vi "Diode_Control_Panel.vi"(11 "IP Address of Remote Device":string="196.254.31.200") -> ()   [LabVIEW 2020]
panel:
  in  "Visualization Tab Control":enum32{"Trace", "Metrics", "None"}(tab)
  out "Diode Trace":waveform(dbl)[](graph)
  out "Reduced Mean Signal, One Point = One Shot":dbl[](graph)
  out "(For your Reference: ) Query Sent to Device":string
  in  "Zero Time":bool
  out "Settable Device Keywords":string[](array[string])
  out "Live Readback Values":string[](array[string])
  in  "Set All":bool
  in  "Set Values\n(Fully empty cells will not be set)":string[](array[string])
  out "Live Responses":string[](array[string])
  out "Non-Settable Device Keywords":string[](array[string])
  in  "Disconnect":bool
  # "Diode Control Panel"
  # "General control panel to facilitate setup of diode, setting times, verifying quality of metrics."
  # "VI Instructions\n\n1. Make sure you know the Device IP Address.\n2. From Windows command prompt, confirm ping to IP address.\n3. Type the correct device IP address into this VI.\n3. Run this VI. *Note:* Only one TCP connection to the device's SCPI-like server can run at a time.\n4. When finished, disconnect safely from the device via the \"Disconnect\" toggle button. (Not the Abort button).\n\nCreated by Scott Feister on July 19, 2022.\nUpdated back panel details July 28, 2022."
  # "1. Resets the trigger count to zero.\n2. Transmits this system's current time."
  # "Settings *ARE NOT SAVED TO DEVICE* and are lost on device reset! Write them down!"
  # "Select the \"None\" tab to help other items update more quickly, and to save network bandwidth."
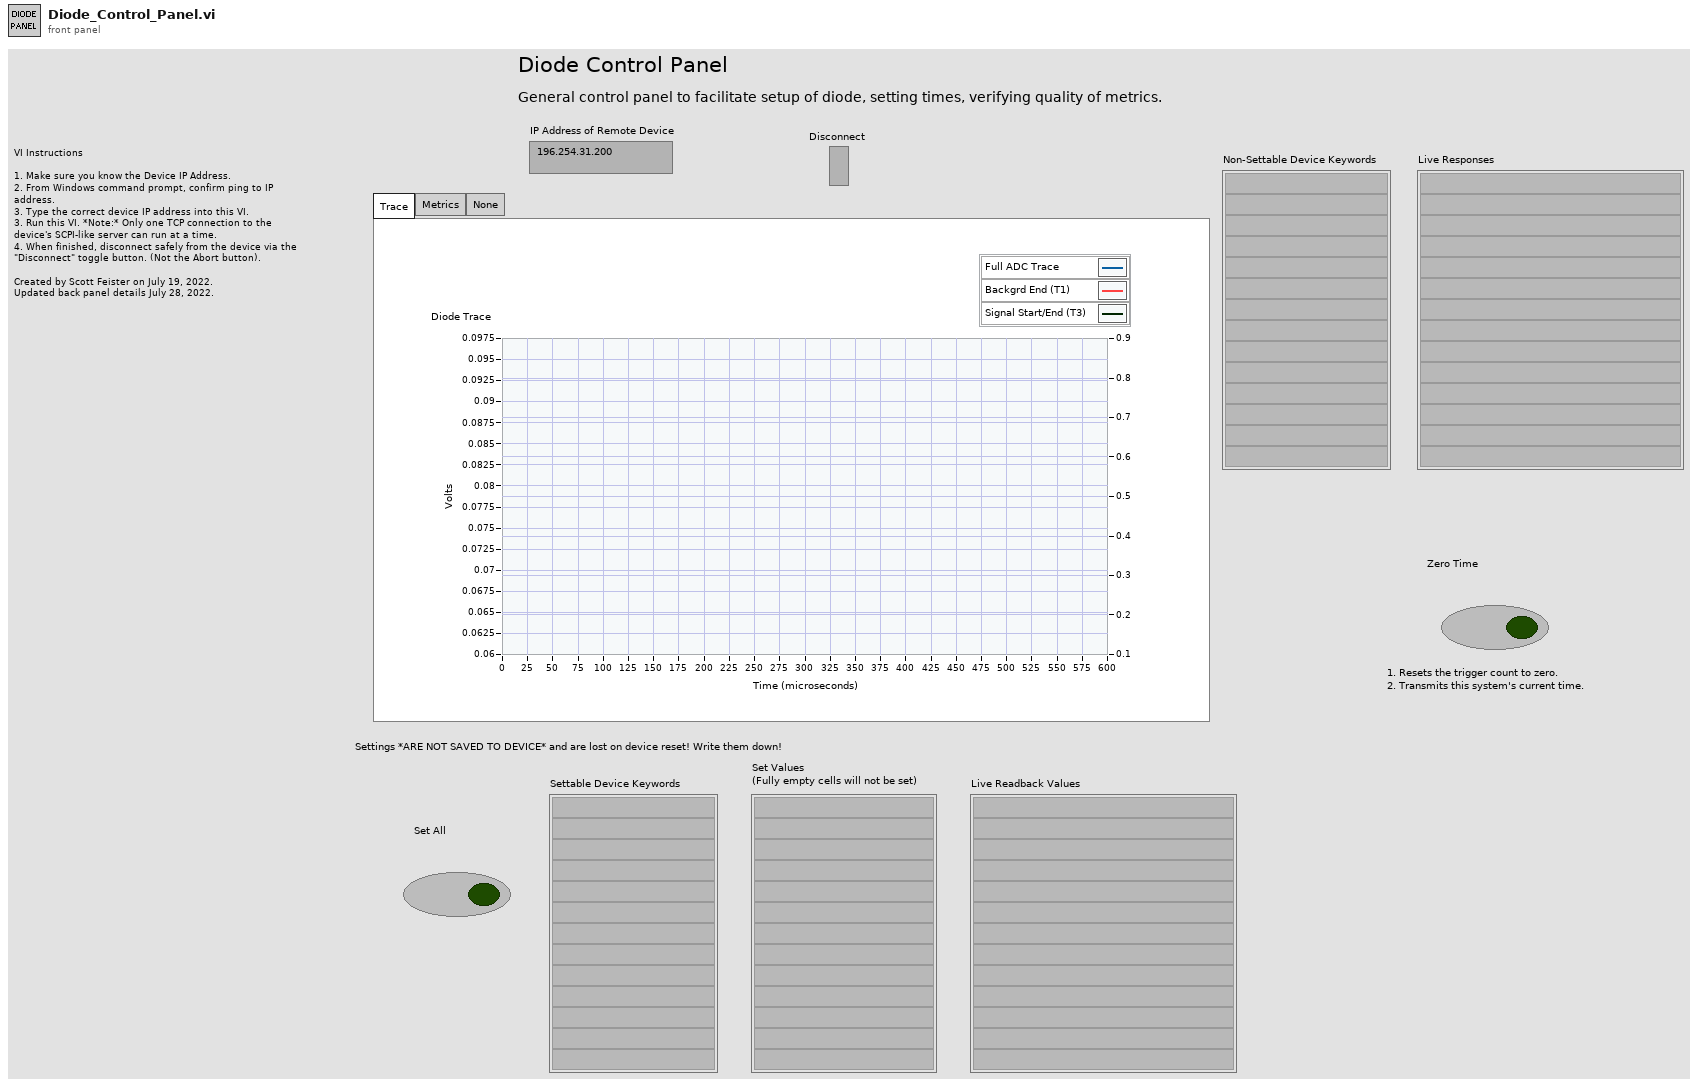
[diagram p1: front panel]
types:
  T1 = typedef "DDAQ-Keyword.ctl" = cluster{"Keyword":string, "Gettable":bool, "Settable":bool, "Is Array":bool, "Data Type":string, "Description":string}
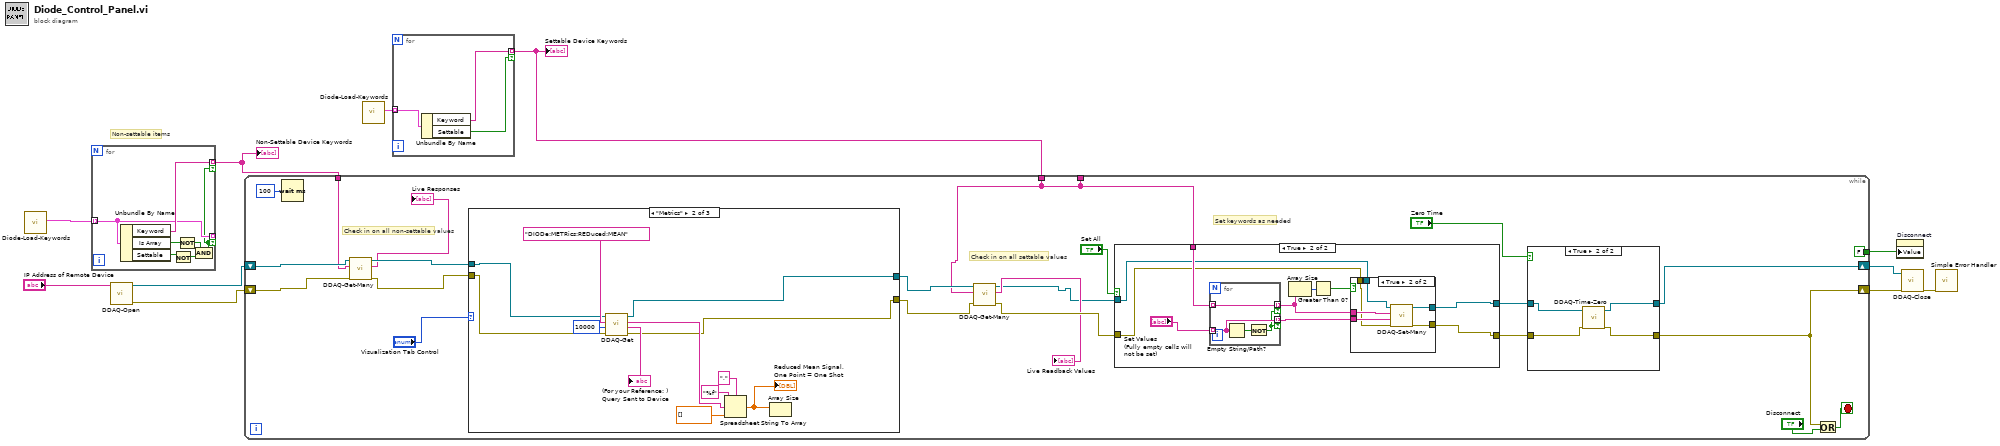
[diagram p0: block diagram]
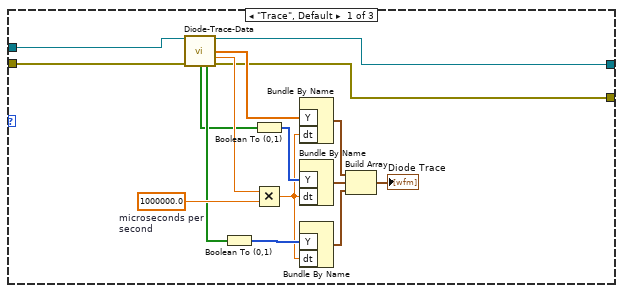
[diagram p2: hidden frame]
diagram:
  # "Non-settable items"
  n1 = call "Diode-Load-Keywords.vi"() -> ("Diodes Keywords Array"=w4:T1[])  [unwired: 11 in]
  n2 = for {
    tunnel: w4 -> [w16] mode=indexing
    tunnel: [w18] -> w2 mode=indexing if=w12
    tunnel: [w16] -> _ mode=indexing if=w12
    n3 = Unbundle By Name(w16) -> ("Keyword"=w18:string, "Is Array"=w17:bool, "Settable"=w15:bool)
    n4 = Not(x=w15) -> (.not. x?=w14:bool)
    n5 = Not(x=w17) -> (.not. x?=w13:bool)
    n6 = And(x=w13, y=w14) -> (x .and. y?=w12:bool)
  }
  "Non-Settable Device Keywords" <- w2
  n7 = call "DDAQ-Open.vi"("IP Address of Nucleo Device"="IP Address of Remote Device") -> ("error out"=w10:errorcluster, "connection ID"=w11:refnum<k5>)  [unwired: 8 in, 1 out]
  n8 = call "Diode-Load-Keywords.vi"() -> ("Diodes Keywords Array"=w3:T1[])  [unwired: 11 in]
  n9 = for {
    tunnel: w3 -> [w20] mode=indexing
    tunnel: [w21] -> w1 mode=indexing if=w19
    n10 = Unbundle By Name(w20) -> ("Keyword"=w21:string, "Settable"=w19:bool)
  }
  "Settable Device Keywords" <- w1
  n11 = while {
    shift-right: [w36] -> w9
    shift-left: w11 -> [w33]
    shift-right: [w35] -> w8
    shift-left: w10 -> [w32]
    tunnel: [FALSE] -> w6
    tunnel: [w22] -> _
    tunnel: w2 -> [w28]
    tunnel: w1 -> [w22]
    stop <- w41 stop-if-true
    # "Set keywords as needed"
    # "Check in on all settable values"
    # "Check in on all non-settable values"
    n12 = Wait (ms)(milliseconds to wait=u32 100) -> ()  [unwired: 1 out]
    n13 = call "DDAQ-Get-Many.vi"("error in (no error)"=w32, "SCPI-like Keywords (leave off question marks)"=w28, "connection ID"=w33) -> ("error out"=w31:errorcluster, "Responses"=→"Live Responses":string[], "connection ID out"=w30:refnum<k5>)  [unwired: 4 in, 2 out]
    n14 = case shown="\"Metrics\"" "Visualization Tab Control" {
      tunnel: w30 -> [w60 w64 w74]
      tunnel: w31 -> [w59 w63 w73]
      tunnel: [w46 w61 w74] -> w27
      tunnel: [w45 w62 w73] -> w26
      frame "Trace", Default {
        w56 = 1000000.0  # microseconds per second
        n15 = call "Diode-Trace-Data.vi"("connection ID"=w60, "error in (no error)"=w59) -> ("connection ID out"=w46:refnum<k5>, "Trace (Volts)"=w58:dbl[], "dt"=w57:dbl, "Background Mask Array"=w47:bool[], "Signal Mask Array"=w48:bool[], "error out"=w45:errorcluster)  [unwired: 5 in, 3 out]
        n16 = Boolean To (0,1)(Boolean=w48) -> (0, 1=w54:i16[])
        n17 = Boolean To (0,1)(Boolean=w47) -> (0, 1=w55:i16[])
        n18 = Multiply(x=w57, y=w56) -> (x*y=w53:dbl)
        n19 = Bundle By Name("Y"=w58, "dt"=w53) -> (w50:waveform(dbl))  [unwired: 1 in]
        n20 = Bundle By Name("Y"=w55, "dt"=w53) -> (w52:waveform(i16))  [unwired: 1 in]
        n21 = Bundle By Name("Y"=w54, "dt"=w53) -> (w51:waveform(i16))  [unwired: 1 in]
        n22 = Build Array(w50, w52, w51) -> (→"Diode Trace":waveform(dbl)[])
      }
      frame "Metrics" {
        n23 = call "DDAQ-Get.vi"("error in (no error)"=w63, "max bytes to read (10000)"=10000 ("max bytes to read (500)"), "SCPI-like Keyword (leave off question mark)"="DIODe:METRics:REDuced:MEAN" ("Diode Keyword (leave off question mark)"), "connection ID"=w64) -> ("error out"=w62:errorcluster, "Query"=→"(For your Reference: ) Query Sent to Device":string, "Response"=w71:string, "connection ID out"=w61:refnum<k5>)  [unwired: 3 in, 1 out]
        n24 = Spreadsheet String To Array(delimiter (Tab)=",", format string="%f", spreadsheet string=w71, array type (2D Dbl)=dbl[] []) -> (array=w72:dbl[])
        "Reduced Mean Signal, One Point = One Shot" <- w72
        n25 = Array Size(array=w72) -> ()  [unwired: 1 out]
      }
      frame "None" {
      }
    }
    n26 = call "DDAQ-Get-Many.vi"("error in (no error)"=w26, "SCPI-like Keywords (leave off question marks)"=w22, "connection ID"=w27) -> ("error out"=w25:errorcluster, "Responses"=→"Live Readback Values":string[], "connection ID out"=w23:refnum<k5>)  [unwired: 4 in, 2 out]
    n27 = case shown="True" "Set All" {
      tunnel: w22 -> [_ w91]
      tunnel: w23 -> [w81 w87]
      tunnel: w25 -> [w82 w86]
      tunnel: [w82 w83] -> w37
      tunnel: [w81 w84] -> w38
      frame False {
      }
      frame True {
        n28 = for {
          tunnel: "Set Values\n(Fully empty cells will not be set)" -> [w102] mode=indexing
          tunnel: w91 -> [w103] mode=indexing
          tunnel: [w103] -> w89 mode=indexing if=w101
          tunnel: [w102] -> w88 mode=indexing if=w101
          n29 = Empty String/Path?(string/path=w102) -> (empty?=w104:bool)
          n30 = Not(x=w104) -> (.not. x?=w101:bool)
        }
        n31 = Array Size(array=w89) -> (size(s)=w90:i32)
        n32 = Greater Than 0?(x=w90) -> (x > 0?=w85:bool)
        n33 = case shown="True" w85 {
          tunnel: w89 -> [_ w100]
          tunnel: w88 -> [_ w99]
          tunnel: w87 -> [w94 w98]
          tunnel: w86 -> [w93 w97]
          tunnel: [w94 w96] -> w84
          tunnel: [w93 w95] -> w83
          frame False {
          }
          frame True {
            n34 = call "DDAQ-Set-Many.vi"("error in (no error)"=w97, "Set Values"=w99, "SCPI-like Keywords (leave off space, value)"=w100, "connection ID"=w98) -> ("error out"=w95:errorcluster, "connection ID out"=w96:refnum<k5>)  [unwired: 5 in, 1 out]
          }
        }
      }
    }
    n35 = case shown="True" "Zero Time" {
      tunnel: w38 -> [w75 w80]
      tunnel: [w76 w77] -> w35
      tunnel: w37 -> [w76 w78]
      tunnel: [w75 w79] -> w36
      frame False {
      }
      frame True {
        n36 = call "DDAQ-Time-Zero.vi"("error in (no error)"=w78, "connection ID"=w80) -> ("error out"=w77:errorcluster, "connection ID out"=w79:refnum<k5>)  [unwired: 8 in]
      }
    }
    n37 = Or(x=w35, y="Disconnect") -> (x .or. y?=w41:bool)
  }
  n38 = property on="Disconnect" class="Bool (strict)"("Value"=w6) -> ()  [unwired: 2 in, 2 out]
  n39 = call "DDAQ-Close.vi"("error in (no error)"=w8, "connection ID"=w9) -> ("error out"=w7:errorcluster)  [unwired: 8 in, 1 out]
  n40 = call <vilib>:"Simple Error Handler.vi"("error in (no error)"=w7) -> ()  [unwired: 4 in, 5 out]
